vi "Get Channel (Blue).vi"(8 "error in (no error)":errorcluster, 10 "Greyscale Image Destination in":T1, 11 "ARGB Image Source in":T2) -> (0 "error out":errorcluster, 3 "Greyscale Image Destination":T1)   [LabVIEW 2020, in "image.lvlib"]
doc: "Get the Blue channel as a single-channel Greyscale Image. The Destination Image will be sized to fit the Source Image."
uses:
  image.lvlib
  Greyscale Image.ctl
  ARGB Image.ctl
  ExtractOptions.ctl
  <vilib>/Utility/error.llb/Error Cluster From Error Code.vi
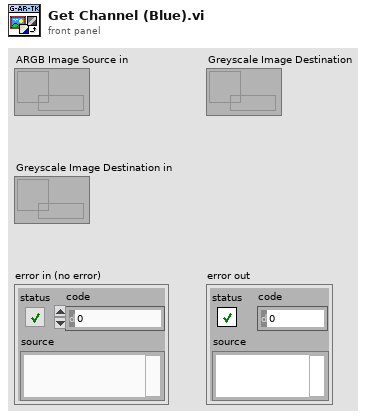
[diagram p1: front panel]
types:
  T1 = typedef "image.lvlib/Greyscale Image.ctl" = refnum<data-value>
  T2 = typedef "image.lvlib/ARGB Image.ctl" = refnum<data-value>
  T3 = typedef "image.lvlib/ExtractOptions.ctl" = enum8{"Blue", "Green", "Red", "Alpha", "Greyscale"}
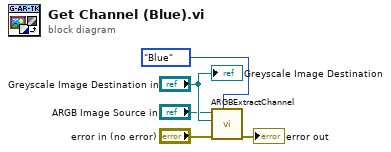
[diagram p0: block diagram]
diagram:
  n1 = call "ARGBExtractChannel.vi"("ExtractOperation"=ExtractOptions."Blue" ("Extract_Operation"), "error in (no error)"="error in (no error)", "Greyscale Image Destination in"="Greyscale Image Destination in", "ARGB Image Source in"="ARGB Image Source in") -> ("error out"=→"error out":errorcluster)  [unwired: 7 in]
  "Greyscale Image Destination" <- "Greyscale Image Destination in"
